vi "Array Sample1.vi"() -> ()   [LabVIEW 2024]
panel:
  out "Output String Array":string[](array[string])
  in  "Input String Array":string[](array[string])
  out "Array 4":bool[](array[boolean])
  in  "Array 3":bool[](array[boolean])
  out "Array 2":dbl[](array[slide]) scale=0.0..20.0
  in  "Array":dbl[](array[numeric])
  # "Overview:\nArray is used to give multiple elements in one element.\n\nInstructions:\n1. Give the values in the Array elements.\n2. Run the VI."
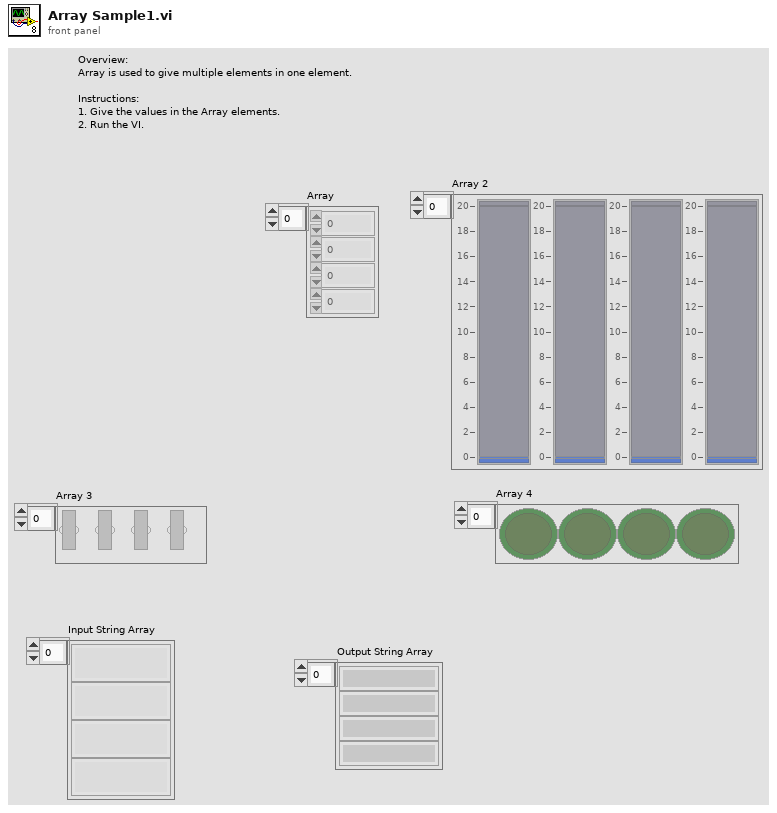
[diagram p1: front panel]
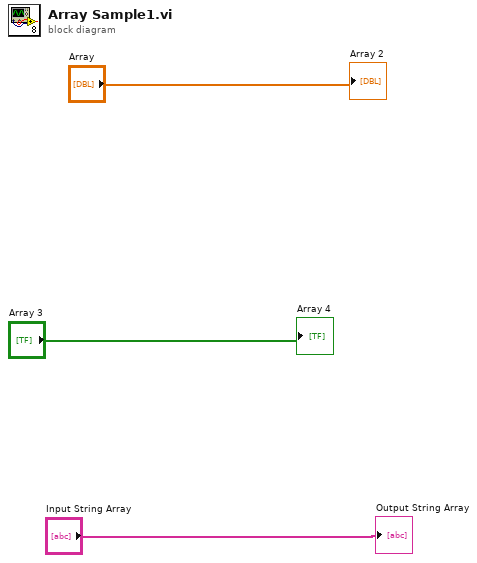
[diagram p0: block diagram]
diagram:
  "Array 2" <- "Array"
  "Array 4" <- "Array 3"
  "Output String Array" <- "Input String Array"
